vi "Constructor_LogRecord.vi"(7 "Level":T1, 8 "Error to log":errorcluster, 9 "Source":string, 10 "Message":string, 11 "LogRecord in":refnum<class "LogRecord.lvclass">) -> (3 "LogRecord out":refnum<class "LogRecord.lvclass">)   [LabVIEW 2024, in "LogRecord.lvclass"]
uses:
  LogRecord.lvclass
  LogRecord.lvclass/LogRecord.ctl
  Shared/Level.ctl
  Shared/LoggerShared.lvlib
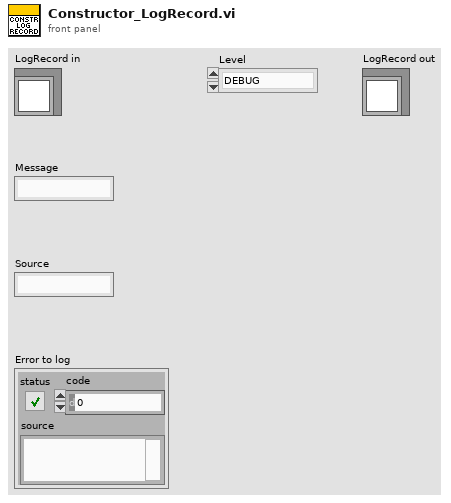
[diagram p1: front panel]
types:
  T1 = typedef "LoggerShared.lvlib/Level.ctl" = enum16{"DEBUG", "INFO", "WARNING", "ERROR", "CRITICAL"}
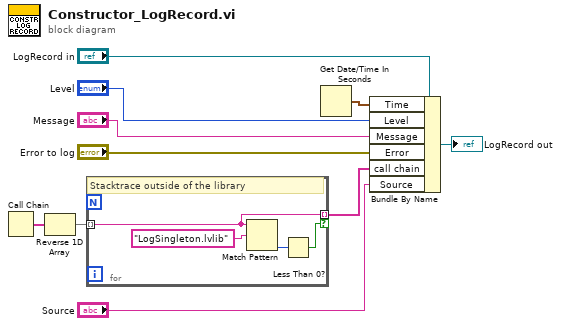
[diagram p0: block diagram]
diagram:
  n1 = Call Chain() -> (call chain=w7:string[])
  n2 = Reverse 1D Array(array=w7) -> (reversed array=w6:string[])
  n3 = for {
    tunnel: w6 -> [w12] mode=indexing
    tunnel: [w12] -> w1 mode=indexing if=w11
    # "Stacktrace outside of the library"
    n4 = Match Pattern(string=w12, regular expression="LogSingleton.lvlib") -> (offset past match=w13:i32)  [unwired: 1 in, 3 out]
    n5 = Less Than 0?(x=w13) -> (x < 0?=w11:bool)
  }
  n6 = Get Date/Time In Seconds() -> (seconds since 1Jan1904=w8:timestamp)
  n7 = Bundle By Name(cluster="LogRecord in", "Time"=w8, "Level"="Level", "Message"="Message", "Error"="Error to log", "call chain"=w1, "Source"="Source") -> (→"LogRecord out":refnum<class "LogRecord.lvclass">)
